vi "波形属性.vi"() -> ()   [LabVIEW 2010]
uses:
  <vilib>/measure/NI_MABase.lvlib
panel:
  out "值":variant[](array[variant])
  out "名称":string[](array[string])
  out "波形输出":waveform(dbl)
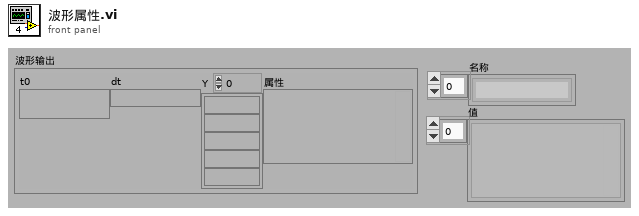
[diagram p1: front panel]
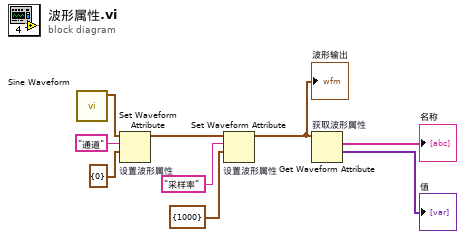
[diagram p0: block diagram]
diagram:
  n1 = call <vilib>:"Sine Waveform.vi"() -> ("signal out"=w5:waveform(dbl))  [unwired: 10 in, 1 out]
  n2 = Set Waveform Attribute "设置波形属性"(5:cluster{i32} {0} ("value"), 6:"通道" ("name"), 7:w5) -> (3:w4:waveform(dbl))  [unwired: 1 in, 2 out]
  n3 = Set Waveform Attribute "设置波形属性"(5:cluster{i32} {1000} ("value"), 6:"采样率" ("name"), 7:w4) -> (3:w3:waveform(dbl))  [unwired: 1 in, 2 out]
  "波形输出" <- w3
  n4 = Get Waveform Attribute "获取波形属性"(7:w3) -> (1:→"值":variant[], 2:→"名称":string[])  [unwired: 3 in, 2 out]
